vi "FusePose.vi"(0 "Lime Vision Valid [t-?]":bool, 1 "Odometry Timestamp (ms)":u32, 2 "Odometry Delta X (in) [t0]":dbl, 3 "Odometry Delta Y (in) [t0]":dbl, 5 "Vision X (in) [t-?]":dbl, 7 "Vision Y (in) [t-?]":dbl, 9 "Vision Timestamp (ms)":u32, 11 "Lemon Vision Valid [t-?]":bool, 12 "Pose Mode":T1(ring)) -> (4 "X (in) [t0]":dbl, 6 "Y (in) [t0]":dbl, 10 "X Odometry Only (in) [t0]":dbl, 15 "Y Odometry Only (in) [t0]":dbl)   [LabVIEW 2023]
doc: "This VI fuses multiple sensing modalities to estimate the robot's current pose."
uses:
  7b9bb9b1-306e-4d3e-b7ed-2eba6d8170c6.vi
  1559d662-8abd-40e9-a5dc-3c53134ee71a.vi
  524daecc-998c-4826-9d6e-2db19cf0bc7c.vi
  GlobalDriverStationData.vi
  GlobalPoseAndTargeting.vi
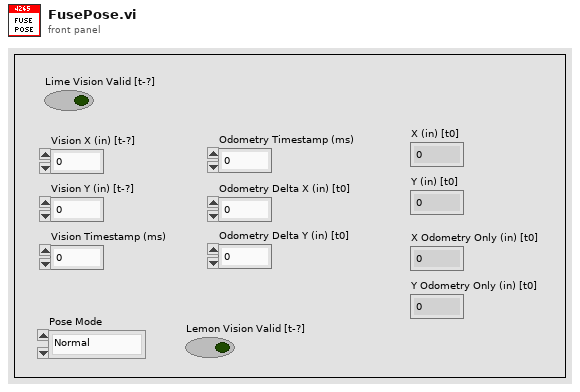
[diagram p1: front panel]
types:
  T1 = enum16{"Normal", "Auto Set", "Reset IMU", "Manual Push", "Init"}
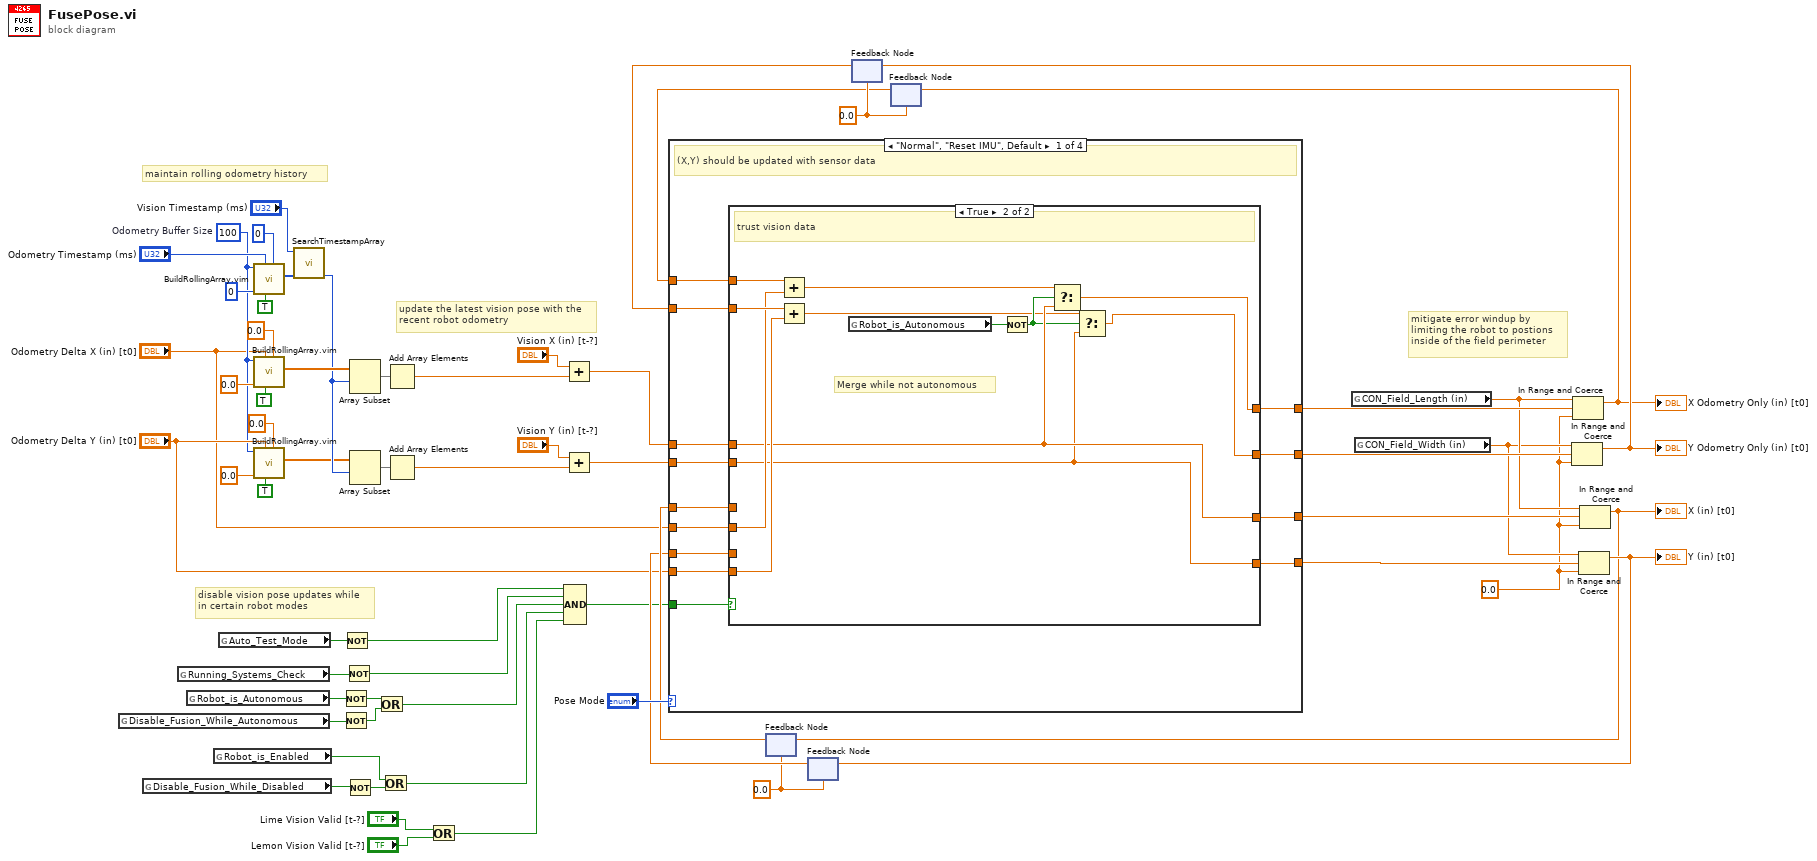
[diagram p0: block diagram]
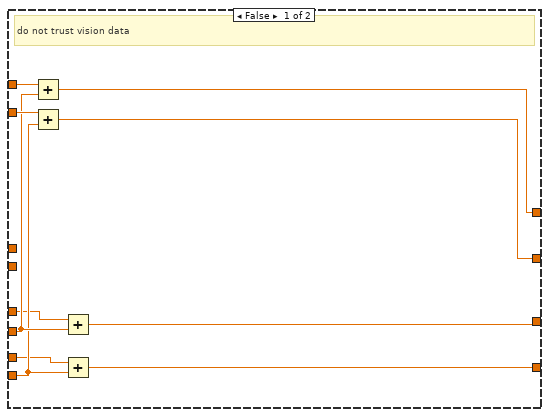
[diagram p2: hidden frame]
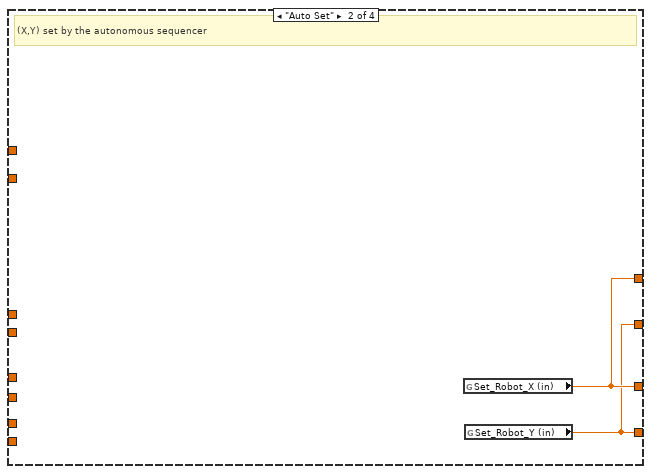
[diagram p3: hidden frame]
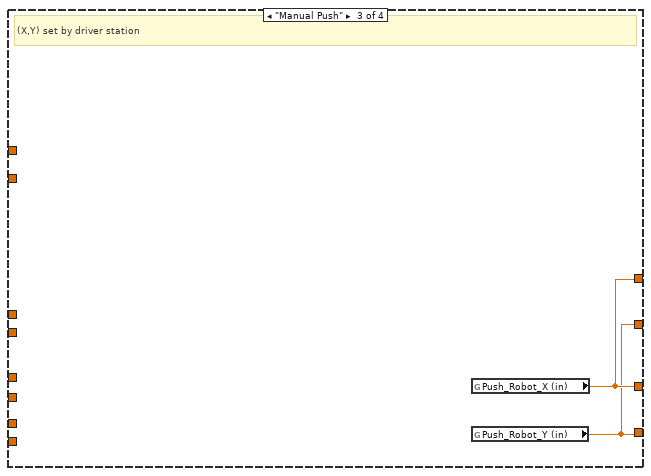
[diagram p4: hidden frame]
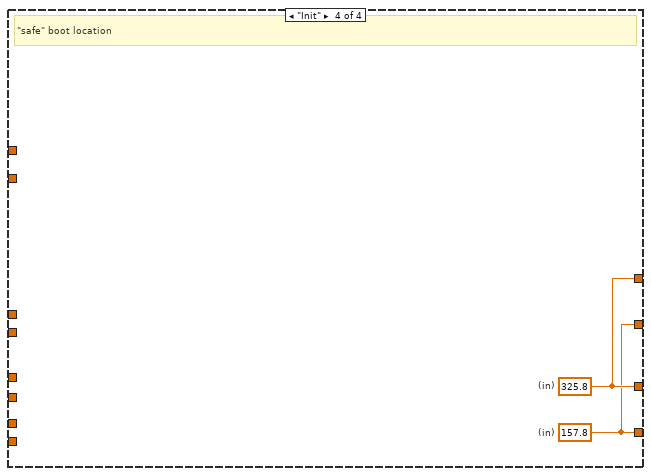
[diagram p5: hidden frame]
diagram:
  w1 = 0.0 ("lower limit")
  w24 = 0.0
  w43 = 0.0
  w21 = 100  # Odometry Buffer Size
  # "disable vision pose updates while\nin certain robot modes"
  # "maintain rolling odometry history"
  # "update the latest vision pose with the\nrecent robot odometry"
  # "mitigate error windup by\nlimiting the robot to postions\ninside of the field perimeter"
  n1 = global read "GlobalDriverStationData.vi" "Disable_Fusion_While_Autonomous"() -> (w33:bool)
  n2 = global read "GlobalDriverStationData.vi" "Disable_Fusion_While_Disabled"() -> (w36:bool)
  n3 = global read "GlobalDriverStationData.vi" "Running_Systems_Check"() -> (w15:bool)
  n4 = global read "GlobalDriverStationData.vi" "Robot_is_Autonomous"() -> (w35:bool)
  n5 = global read "GlobalDriverStationData.vi" "Robot_is_Enabled"() -> (w9:bool)
  n6 = global read "GlobalDriverStationData.vi" "Auto_Test_Mode"() -> (w8:bool)
  n7 = call "BuildRollingArray.vim"("Global Additive Update"=0, "Update?"=TRUE, "New Value"="Odometry Timestamp (ms)", "Initial Value"=0, "Number of Elements"=w21) -> ("Current Array"=w57:u32[])  [unwired: 6 in]
  n8 = call "BuildRollingArray.vim"("Global Additive Update"=0.0, "Update?"=TRUE, "New Value"="Odometry Delta X (in) [t0]", "Initial Value"=0.0, "Number of Elements"=w21) -> ("Current Array"=w54:dbl[])  [unwired: 6 in]
  n9 = call "BuildRollingArray.vim"("Global Additive Update"=0.0, "Update?"=TRUE, "New Value"="Odometry Delta Y (in) [t0]", "Initial Value"=0.0, "Number of Elements"=w21) -> ("Current Array"=w49:dbl[])  [unwired: 6 in]
  n10 = call "SearchTimestampArray.vi"("Timestamp Array"=w57, "Search Timestamp"="Vision Timestamp (ms)") -> ("Closest Index"=w50:i32)  [unwired: 8 in, 1 out]
  n11 = Not(x=w35) -> (.not. x?=w34:bool)
  n12 = Not(x=w33) -> (.not. x?=w32:bool)
  n13 = Not(x=w8) -> (.not. x?=w7:bool)
  n14 = Not(x=w15) -> (.not. x?=w14:bool)
  n15 = Not(x=w36) -> (.not. x?=w30:bool)
  n16 = Array Subset(array=w54, index=w50) -> (w55:dbl[])  [unwired: 1 in]
  n17 = Array Subset(array=w49, index=w50) -> (w52:dbl[])  [unwired: 1 in]
  n18 = Or(x=w34, y=w32) -> (x .or. y?=w31:bool)
  n19 = Or(x=w9, y=w30) -> (x .or. y?=w29:bool)
  n20 = Add Array Elements(numeric array=w55) -> (sum=w53:dbl)
  n21 = Add Array Elements(numeric array=w52) -> (sum=w51:dbl)
  n22 = Or(x="Lime Vision Valid [t-?]", y="Lemon Vision Valid [t-?]") -> (x .or. y?=w4:bool)
  n23 = Add(x="Vision X (in) [t-?]", y=w53) -> (x+y=w46:dbl)
  n24 = Add(x="Vision Y (in) [t-?]", y=w51) -> (x+y=w47:dbl)
  n25 = Compound Arithmetic op=AND(w7, w14, w31, w29, w4) -> (w37:bool)
  n26 = feedback #1(w43) -> (w45:dbl)
  n27 = feedback #2(w43) -> (w44:dbl)
  n28 = feedback #3(w24) -> (w22:dbl)
  n29 = feedback #4(w24) -> (w23:dbl)
  n30 = case shown="\"Normal\", \"Reset IMU\", Default" "Pose Mode" {
    tunnel: [w70 w98 w100 w102] -> w12
    tunnel: w45 -> [w74 _ _ _]
    tunnel: "Odometry Delta X (in) [t0]" -> [w73 _ _ _]
    tunnel: w44 -> [w72 _ _ _]
    tunnel: "Odometry Delta Y (in) [t0]" -> [w71 _ _ _]
    tunnel: [w69 w97 w99 w101] -> w13
    tunnel: w37 -> [w68 _ _ _]
    tunnel: w47 -> [w67 _ _ _]
    tunnel: w46 -> [w66 _ _ _]
    tunnel: [w65 w98 w100 w102] -> w17
    tunnel: [w64 w97 w99 w101] -> w19
    tunnel: w23 -> [w63 _ _ _]
    tunnel: w22 -> [w62 _ _ _]
    frame "Normal", "Reset IMU", Default {
      # "(X,Y) should be updated with sensor data"
      n31 = case shown="True" w68 {
        tunnel: w74 -> [w78 _]
        tunnel: w73 -> [w80 w94]
        tunnel: w72 -> [w77 _]
        tunnel: w71 -> [w79 w93]
        tunnel: [w76 w90] -> w70
        tunnel: [w75 w88] -> w69
        tunnel: w67 -> [_ w88]
        tunnel: w66 -> [_ w90]
        tunnel: [w82 w92] -> w65
        tunnel: [w81 w86] -> w64
        tunnel: w63 -> [w84 w96]
        tunnel: w62 -> [w83 w95]
        frame False {
          # "do not trust vision data"
          n32 = Add(x=w84, y=w80) -> (x+y=w82:dbl)
          n33 = Add(x=w83, y=w79) -> (x+y=w81:dbl)
          n34 = Add(x=w78, y=w80) -> (x+y=w76:dbl)
          n35 = Add(x=w77, y=w79) -> (x+y=w75:dbl)
        }
        frame True {
          # "Merge while not autonomous"
          # "trust vision data"
          n36 = Add(x=w96, y=w94) -> (x+y=w91:dbl)
          n37 = Add(x=w95, y=w93) -> (x+y=w87:dbl)
          n38 = global read "GlobalDriverStationData.vi" "Robot_is_Autonomous"() -> (w85:bool)
          n39 = Not(x=w85) -> (.not. x?=w89:bool)
          n40 = Select(t=w91, s=w89, f=w90) -> (s? t:f=w92:dbl)
          n41 = Select(t=w87, s=w89, f=w88) -> (s? t:f=w86:dbl)
        }
      }
    }
    frame "Auto Set" {
      # "(X,Y) set by the autonomous sequencer"
      n42 = global read "GlobalPoseAndTargeting.vi" "Set_Robot_X (in)"() -> (w98:dbl)
      n43 = global read "GlobalPoseAndTargeting.vi" "Set_Robot_Y (in)"() -> (w97:dbl)
    }
    frame "Manual Push" {
      # "(X,Y) set by driver station"
      n44 = global read "GlobalPoseAndTargeting.vi" "Push_Robot_X (in)"() -> (w100:dbl)
      n45 = global read "GlobalPoseAndTargeting.vi" "Push_Robot_Y (in)"() -> (w99:dbl)
    }
    frame "Init" {
      w101 = 157.8  # (in)
      w102 = 325.8  # (in)
      # "\"safe\" boot location"
    }
  }
  n46 = global read "GlobalPoseAndTargeting.vi" "CON_Field_Length (in)"() -> (w3:dbl)
  n47 = global read "GlobalPoseAndTargeting.vi" "CON_Field_Width (in)"() -> (w2:dbl)
  n48 = In Range and Coerce(upper limit=w2, x=w19, lower limit=w1) -> (coerced(x)=w18:dbl)  [unwired: 1 out]
  "Y Odometry Only (in) [t0]" <- w18
  n49 = feedback-in #3(w18) -> ()
  n50 = In Range and Coerce(upper limit=w3, x=w17, lower limit=w1) -> (coerced(x)=w16:dbl)  [unwired: 1 out]
  "X Odometry Only (in) [t0]" <- w16
  n51 = feedback-in #4(w16) -> ()
  n52 = In Range and Coerce(upper limit=w2, x=w13, lower limit=w1) -> (coerced(x)=w11:dbl)  [unwired: 1 out]
  "Y (in) [t0]" <- w11
  n53 = feedback-in #2(w11) -> ()
  n54 = In Range and Coerce(upper limit=w3, x=w12, lower limit=w1) -> (coerced(x)=w10:dbl)  [unwired: 1 out]
  "X (in) [t0]" <- w10
  n55 = feedback-in #1(w10) -> ()
